vi "RSZVB Configure Calibration Unit Standard.vi"(5 "Port 1 (1)":i32=1, 7 "Port 2 (1)":i32=1, 8 "error in (no error)":errorcluster {"code" format="%.0x"}, 10 "Standard (0: Through)":u16(ring) items=["Through", "Open", "Short", "Match"], 11 "VISA session":refnum<visa-resource-name>) -> (0 "error out":errorcluster {"code" format="%.0x"}, 3 "dup VISA session":refnum<visa-resource-name>)   [LabVIEW 2011]
doc: "This VI defines calibration unit standard.\n\nRemote-control command(s):\n:SYSTem:COMMunicate:AKAL:CONNection THRough | OPEN | SHORt | MATCh,<port_number>{,<port_number>}"
uses:
  _utility/RSZVB Global Data.vi
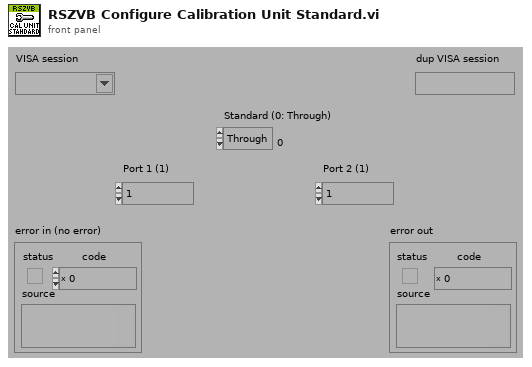
[diagram p1: front panel]
types:
  T1 = cluster{"Error Checking (T: On)":bool, "Installed Options":string[], "Data Valid?":bool, "Ports":i32, "Model":string[], "Option Checking (T: On)":bool}[]
  T2 = cluster{"Error Checking (T: On)":bool, "Installed Options":string[], "Data Valid?":bool, "Ports":i32, "Model":string[], "Option Checking (T: On)":bool}
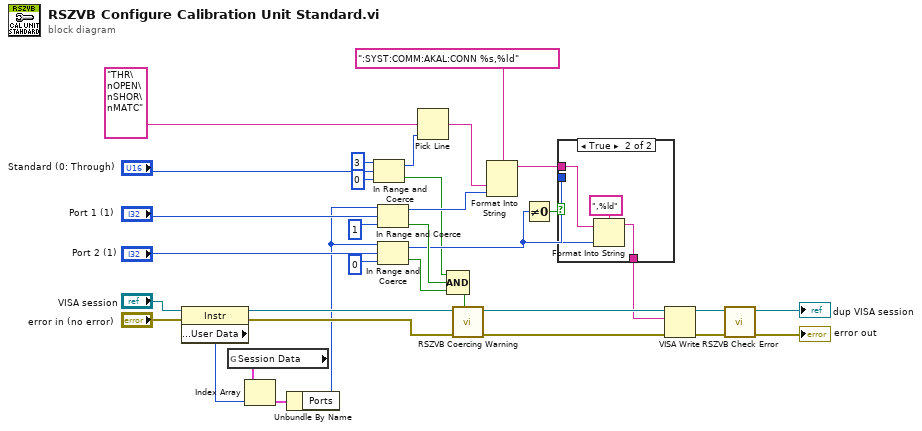
[diagram p0: block diagram]
diagram:
  n1 = property class="Instr"(reference="VISA session", error in="error in (no error)") -> (reference out=w27:refnum<visa-resource-name>, error out=w28:errorcluster, "General Settings:User Data"=w29:u32)
  n2 = global read "RSZVB Global Data.vi" "Session Data"() -> (w30:T1)
  n3 = Index Array(array=w30, index=w29) -> (element=w31:T2)
  n4 = Unbundle By Name(w31) -> ("Ports"=w11:i32)
  n5 = In Range and Coerce(upper limit=u16 3, x="Standard (0: Through)", lower limit=u16 0) -> (coerced(x)=w5:u16, In Range?=w8:bool)
  n6 = In Range and Coerce(upper limit=w11, x="Port 1 (1)", lower limit=1) -> (coerced(x)=w23:i32, In Range?=w22:bool)
  n7 = In Range and Coerce(upper limit=w11, x="Port 2 (1)", lower limit=0) -> (coerced(x)=w17:i32, In Range?=w21:bool)
  n8 = Pick Line(multi-line string="THR\nOPEN\nSHOR\nMATC", line index=w5) -> (output string=w4:string)  [unwired: 1 in]
  n9 = Compound Arithmetic op=AND(w8, w22, w21) -> (w32:bool)
  n10 = call "RSZVB Coercing Warning.vi"("In Range?"=w32, "error in (no error)"=w28, "VISA session"=w27) -> ("error out"=w33:errorcluster, "dup VISA session"=w34:refnum<visa-resource-name>)  [unwired: 7 in]
  n11 = Format Into String(format string=":SYST:COMM:AKAL:CONN %s,%ld", w4, w23) -> (resulting string=w18:string)  [unwired: 2 in, 1 out]
  n12 = Not Equal To 0?(x=w17) -> (x != 0?=w19:bool)
  n13 = case shown="True" w19 {
    tunnel: w18 -> [w35 w39]
    tunnel: w17 -> [_ w37]
    tunnel: [w35 w36] -> w3
    frame False {
    }
    frame True {
      n14 = Format Into String(format string=",%ld", initial string=w39, w37) -> (resulting string=w36:string)  [unwired: 1 in, 1 out]
    }
  }
  n15 = VISA Write(VISA resource name=w34, write buffer=w3, error in (no error)=w33) -> (VISA resource name out=w16:refnum<visa-resource-name>, error out=w15:errorcluster)  [unwired: 1 out]
  n16 = call "RSZVB Check Error.vi"("error in (no error)"=w15, "VISA session"=w16) -> ("error out"=→"error out":errorcluster, "dup VISA session"=→"dup VISA session":refnum<visa-resource-name>)  [unwired: 8 in]
